vi "Test Child Method.vi"(8 "error in (no error)":errorcluster, 11 "Test Case Test Double Child in":refnum<class "Test Case Test Double Child.lvclass">) -> (0 "error out":errorcluster, 3 "Test Case Test Double Child out":refnum<class "Test Case Test Double Child.lvclass">)   [LabVIEW 2020, in "Test Case Test Double Child.lvclass"]
uses:
  Test Case Test Double/Test Case Test Double Child.lvclass
  Test Case Test Double/Test Case Test Double Child.lvclass/Test Case Test Double Child.ctl
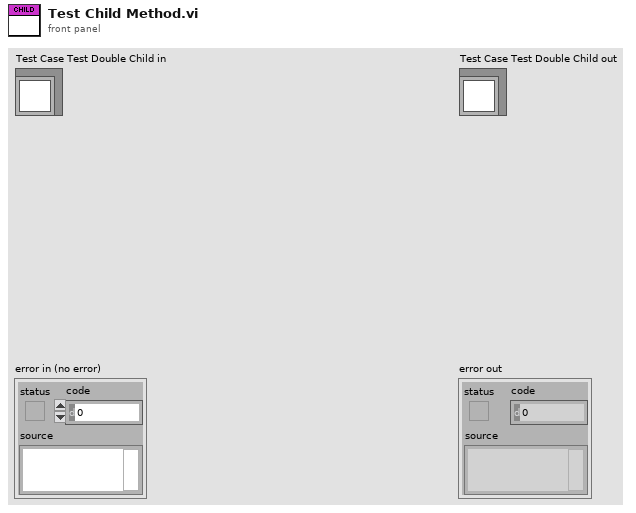
[diagram p1: front panel]
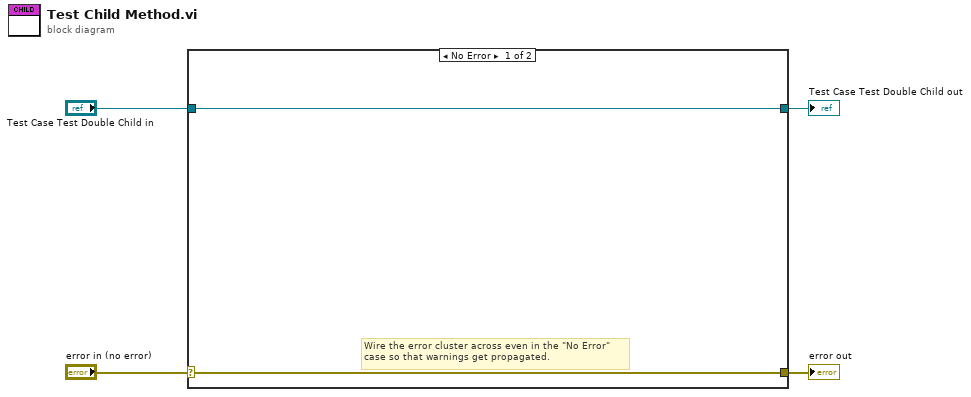
[diagram p0: block diagram]
diagram:
  n1 = case shown="No Error" "error in (no error)" {
    selector: "error in (no error)" -> [w5 w8]
    tunnel: [w5 w8] -> w3
    tunnel: [w6 w7] -> w1
    tunnel: "Test Case Test Double Child in" -> [w6 w7]
    frame No Error {
      # "Wire the error cluster across even in the \"No Error\"\ncase so that warnings get propagated."
    }
    frame Error {
    }
  }
  "error out" <- w3
  "Test Case Test Double Child out" <- w1
